vi "v2.0_fulopbence_plc_mitsubishi_fenyjatek.vi"() -> ()   [LabVIEW 2024]
panel:
  out "Y5":bool
  out "Y4":bool
  out "Y3":bool
  out "Y2":bool
  out "Y1":bool
  out "Y0":bool
  in  "S3":bool
  in  "S2":bool
  in  "S1":bool
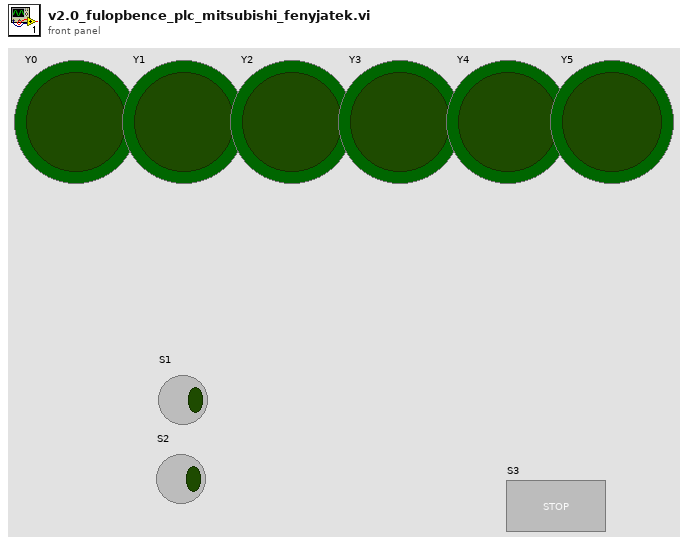
[diagram p1: front panel]
types:
  T1 = enum8{"Enabled", "Disabled", "Disabled and Grayed Out"}
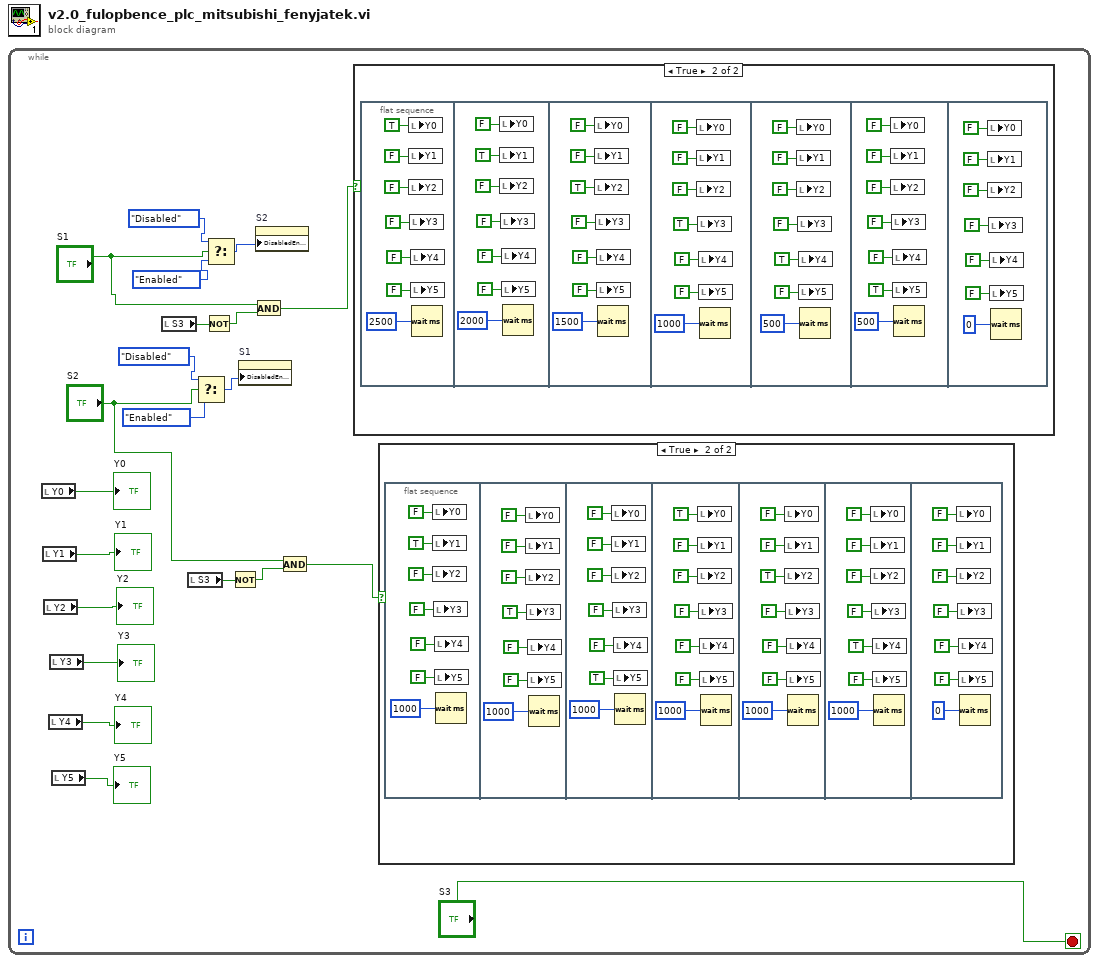
[diagram p0: block diagram]
diagram:
  n1 = while {
    stop <- "S3" stop-if-true
    n2 = local read "Y0"() -> (→"Y0":bool)
    n3 = local read "Y1"() -> (→"Y1":bool)
    n4 = local read "Y2"() -> (→"Y2":bool)
    n5 = local read "Y4"() -> (→"Y4":bool)
    n6 = local read "Y3"() -> (→"Y3":bool)
    n7 = local read "Y5"() -> (→"Y5":bool)
    n8 = local read "S3"() -> (w7:bool)
    n9 = local read "S3"() -> (w4:bool)
    n10 = Select(t=T1."Disabled" ("Disabled"), s="S2", f=T1."Enabled") -> (s? t:f=w21:T1)
    n11 = Not(x=w7) -> (.not. x?=w6:bool)
    n12 = Select(t=T1."Disabled" ("Disabled"), s="S1", f=T1."Enabled") -> (s? t:f=w20:T1)
    n13 = Not(x=w4) -> (.not. x?=w5:bool)
    n14 = property on="S1" class="Bool (strict)"("DisabledEnum"=w21) -> ()  [unwired: 2 in, 2 out]
    n15 = And(x="S1", y=w6) -> (x .and. y?=w8:bool)
    n16 = property on="S2" class="Bool (strict)"("DisabledEnum"=w20) -> ()  [unwired: 2 in, 2 out]
    n17 = And(x="S2", y=w5) -> (x .and. y?=w2:bool)
    n18 = case shown="True" w8 {
      frame False {
      }
      frame True {
        n19 = flat-sequence {
          frame #0 {
            n20 = local write "Y0"(TRUE ("Y0")) -> ()
            n21 = local write "Y1"(FALSE ("Y1")) -> ()
            n22 = local write "Y2"(FALSE ("Y2")) -> ()
            n23 = local write "Y3"(FALSE ("Y3")) -> ()
            n24 = local write "Y4"(FALSE ("Y4")) -> ()
            n25 = local write "Y5"(FALSE ("Y5")) -> ()
            n26 = Wait (ms)(milliseconds to wait=u32 2500) -> ()  [unwired: 1 out]
          }
          frame #1 {
            n27 = local write "Y0"(FALSE ("Y0")) -> ()
            n28 = local write "Y1"(TRUE ("Y1")) -> ()
            n29 = local write "Y2"(FALSE ("Y2")) -> ()
            n30 = local write "Y3"(FALSE ("Y3")) -> ()
            n31 = local write "Y4"(FALSE ("Y4")) -> ()
            n32 = local write "Y5"(FALSE ("Y5")) -> ()
            n33 = Wait (ms)(milliseconds to wait=u32 2000) -> ()  [unwired: 1 out]
          }
          frame #2 {
            n34 = local write "Y0"(FALSE ("Y0")) -> ()
            n35 = local write "Y1"(FALSE ("Y1")) -> ()
            n36 = local write "Y2"(TRUE ("Y2")) -> ()
            n37 = local write "Y3"(FALSE ("Y3")) -> ()
            n38 = local write "Y4"(FALSE ("Y4")) -> ()
            n39 = local write "Y5"(FALSE ("Y5")) -> ()
            n40 = Wait (ms)(milliseconds to wait=u32 1500) -> ()  [unwired: 1 out]
          }
          frame #3 {
            n41 = local write "Y0"(FALSE ("Y0")) -> ()
            n42 = local write "Y1"(FALSE ("Y1")) -> ()
            n43 = local write "Y2"(FALSE ("Y2")) -> ()
            n44 = local write "Y3"(TRUE ("Y3")) -> ()
            n45 = local write "Y4"(FALSE ("Y4")) -> ()
            n46 = local write "Y5"(FALSE ("Y5")) -> ()
            n47 = Wait (ms)(milliseconds to wait=u32 1000) -> ()  [unwired: 1 out]
          }
          frame #4 {
            n48 = local write "Y0"(FALSE ("Y0")) -> ()
            n49 = local write "Y1"(FALSE ("Y1")) -> ()
            n50 = local write "Y2"(FALSE ("Y2")) -> ()
            n51 = local write "Y3"(FALSE ("Y3")) -> ()
            n52 = local write "Y4"(TRUE ("Y4")) -> ()
            n53 = local write "Y5"(FALSE ("Y5")) -> ()
            n54 = Wait (ms)(milliseconds to wait=u32 500) -> ()  [unwired: 1 out]
          }
          frame #5 {
            n55 = local write "Y0"(FALSE ("Y0")) -> ()
            n56 = local write "Y1"(FALSE ("Y1")) -> ()
            n57 = local write "Y2"(FALSE ("Y2")) -> ()
            n58 = local write "Y3"(FALSE ("Y3")) -> ()
            n59 = local write "Y4"(FALSE ("Y4")) -> ()
            n60 = local write "Y5"(TRUE ("Y5")) -> ()
            n61 = Wait (ms)(milliseconds to wait=u32 500) -> ()  [unwired: 1 out]
          }
          frame #6 {
            n62 = local write "Y0"(FALSE ("Y0")) -> ()
            n63 = local write "Y1"(FALSE ("Y1")) -> ()
            n64 = local write "Y2"(FALSE ("Y2")) -> ()
            n65 = local write "Y3"(FALSE ("Y3")) -> ()
            n66 = local write "Y4"(FALSE ("Y4")) -> ()
            n67 = local write "Y5"(FALSE ("Y5")) -> ()
            n68 = Wait (ms)(milliseconds to wait=u32 0) -> ()  [unwired: 1 out]
          }
        }
      }
    }
    n69 = case shown="True" w2 {
      frame False {
      }
      frame True {
        n70 = flat-sequence {
          frame #0 {
            n71 = local write "Y0"(FALSE ("Y0")) -> ()
            n72 = local write "Y1"(TRUE ("Y1")) -> ()
            n73 = local write "Y2"(FALSE ("Y2")) -> ()
            n74 = local write "Y3"(FALSE ("Y3")) -> ()
            n75 = local write "Y4"(FALSE ("Y4")) -> ()
            n76 = local write "Y5"(FALSE ("Y5")) -> ()
            n77 = Wait (ms)(milliseconds to wait=u32 1000) -> ()  [unwired: 1 out]
          }
          frame #1 {
            n78 = local write "Y0"(FALSE ("Y0")) -> ()
            n79 = local write "Y1"(FALSE ("Y1")) -> ()
            n80 = local write "Y2"(FALSE ("Y2")) -> ()
            n81 = local write "Y3"(TRUE ("Y3")) -> ()
            n82 = local write "Y4"(FALSE ("Y4")) -> ()
            n83 = local write "Y5"(FALSE ("Y5")) -> ()
            n84 = Wait (ms)(milliseconds to wait=u32 1000) -> ()  [unwired: 1 out]
          }
          frame #2 {
            n85 = local write "Y0"(FALSE ("Y0")) -> ()
            n86 = local write "Y1"(FALSE ("Y1")) -> ()
            n87 = local write "Y2"(FALSE ("Y2")) -> ()
            n88 = local write "Y3"(FALSE ("Y3")) -> ()
            n89 = local write "Y4"(FALSE ("Y4")) -> ()
            n90 = local write "Y5"(TRUE ("Y5")) -> ()
            n91 = Wait (ms)(milliseconds to wait=u32 1000) -> ()  [unwired: 1 out]
          }
          frame #3 {
            n92 = local write "Y0"(TRUE ("Y0")) -> ()
            n93 = local write "Y1"(FALSE ("Y1")) -> ()
            n94 = local write "Y2"(FALSE ("Y2")) -> ()
            n95 = local write "Y3"(FALSE ("Y3")) -> ()
            n96 = local write "Y4"(FALSE ("Y4")) -> ()
            n97 = local write "Y5"(FALSE ("Y5")) -> ()
            n98 = Wait (ms)(milliseconds to wait=u32 1000) -> ()  [unwired: 1 out]
          }
          frame #4 {
            n99 = local write "Y0"(FALSE ("Y0")) -> ()
            n100 = local write "Y1"(FALSE ("Y1")) -> ()
            n101 = local write "Y2"(TRUE ("Y2")) -> ()
            n102 = local write "Y3"(FALSE ("Y3")) -> ()
            n103 = local write "Y4"(FALSE ("Y4")) -> ()
            n104 = local write "Y5"(FALSE ("Y5")) -> ()
            n105 = Wait (ms)(milliseconds to wait=u32 1000) -> ()  [unwired: 1 out]
          }
          frame #5 {
            n106 = local write "Y0"(FALSE ("Y0")) -> ()
            n107 = local write "Y1"(FALSE ("Y1")) -> ()
            n108 = local write "Y2"(FALSE ("Y2")) -> ()
            n109 = local write "Y3"(FALSE ("Y3")) -> ()
            n110 = local write "Y4"(TRUE ("Y4")) -> ()
            n111 = local write "Y5"(FALSE ("Y5")) -> ()
            n112 = Wait (ms)(milliseconds to wait=u32 1000) -> ()  [unwired: 1 out]
          }
          frame #6 {
            n113 = local write "Y0"(FALSE ("Y0")) -> ()
            n114 = local write "Y1"(FALSE ("Y1")) -> ()
            n115 = local write "Y2"(FALSE ("Y2")) -> ()
            n116 = local write "Y3"(FALSE ("Y3")) -> ()
            n117 = local write "Y4"(FALSE ("Y4")) -> ()
            n118 = local write "Y5"(FALSE ("Y5")) -> ()
            n119 = Wait (ms)(milliseconds to wait=u32 0) -> ()  [unwired: 1 out]
          }
        }
      }
    }
  }
